vi "p1.vi"() -> ()   [LabVIEW 2025, in "d1.lvlib"]
uses:
  d1.lvlib
  AOC/AOC.lvlib
panel:
  in  "Example":string="L68\nL30\nR48\nL5\nR60\nL55\nL1\nL99\nR14\nL82"
  in  "Example?":bool
  out "Answer":i64=55607
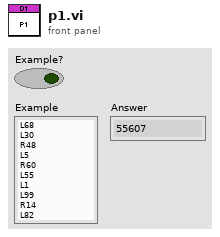
[diagram p1: front panel]
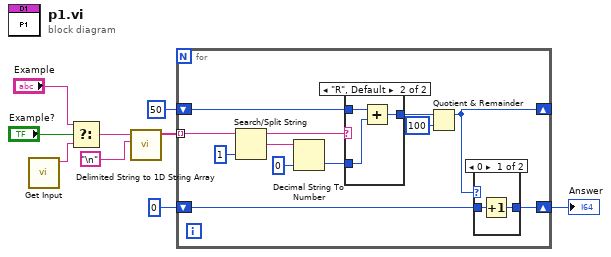
[diagram p0: block diagram]
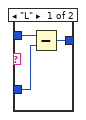
[diagram p3: hidden frame]
diagram:
  n1 = call "Get Input.vi"() -> ("Input"=w8:string)  [unwired: 11 in]
  n2 = Select(t="Example", s="Example?", f=w8) -> (s? t:f=w6:string)
  n3 = call <vilib>:"Delimited String to 1D String Array.vi"("delimiter"="\n", "delimited string"=w6) -> ("string array"=w4:string[])  [unwired: 9 in]
  n4 = for {
    tunnel: w4 -> [w21] mode=indexing
    shift-right: [w10] -> _
    shift-left: i64 50 ("Answer") -> [w19]
    shift-right: [w11] -> w1
    shift-left: i64 0 ("Answer") -> [w12]
    n5 = Search/Split String(string=w21, offset (0)=1) -> (substring before match=w17:string, match + rest of string=w16:string)  [unwired: 1 in, 1 out]
    n6 = Decimal String To Number(string=w16, default (0L)=i64 0 ("default (0 I32)")) -> (number=w15:i64)  [unwired: 1 in, 1 out]
    n7 = case shown="\"R\", Default" w17 {
      tunnel: w19 -> [w27 w30]
      tunnel: [w26 w29] -> w18
      tunnel: w15 -> [w25 w28]
      frame "L" {
        n8 = Subtract(x=w27, y=w25) -> (x-y=w26:i64)
      }
      frame "R", Default {
        n9 = Add(x=w30, y=w28) -> (x+y=w29:i64)
      }
    }
    n10 = Quotient & Remainder(x=w18, y=i64 100) -> (x-y*floor(x/y)=w10:i64)  [unwired: 1 out]
    n11 = case shown="0" w10 {
      tunnel: w12 -> [w23 w24]
      tunnel: [w22 w24] -> w11
      frame 0 {
        n12 = Increment(x=w23) -> (x+1=w22:i64)
      }
      frame Default {
      }
    }
  }
  "Answer" <- w1
